vi "Set Flags.vi"(8 "error in":errorcluster, 10 "Flags":u32 format="%.0x", 11 "Object Entry in":refnum<class "Object Entry.lvclass">) -> (0 "error out":errorcluster, 3 "Object Entry out":refnum<class "Object Entry.lvclass">)   [LabVIEW 2020, in "CANopen.lvlib" / "Object Entry.lvclass"]
uses:
  Object Entry.lvclass
  Object Entry.lvclass/Object Entry.ctl
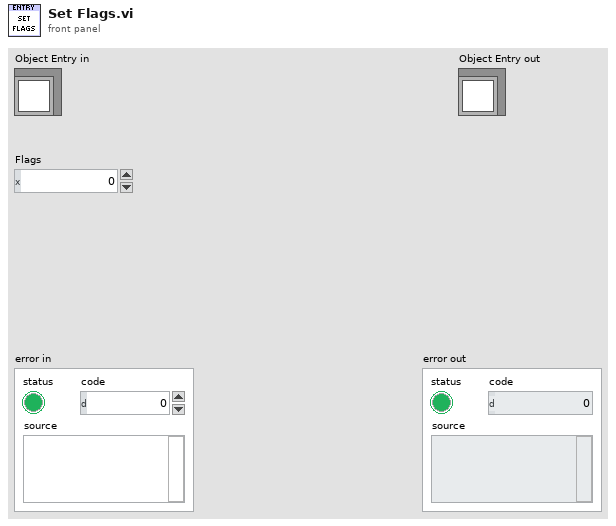
[diagram p1: front panel]
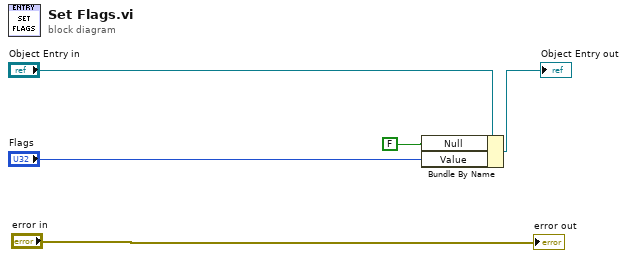
[diagram p0: block diagram]
diagram:
  n1 = Bundle By Name(cluster="Object Entry in", "Null"=FALSE ("Flags.Null"), "Value"="Flags") -> (→"Object Entry out":refnum<class "Object Entry.lvclass">)
  "error out" <- "error in"
